vi "FRCts20_WebMethods_Home_Convert.vi"(8 "error in (no error)":errorcluster, 11 "EventRoot Out":T4) -> (0 "error out":errorcluster, 3 "Events":T1)   [LabVIEW 2014, in "FRCts20_WebMethods.lvlib"]
uses:
  FRCts20_WebMethods.lvlib
  Web Method Public Interface/FRCts20_WebMethods_ctl_teamIdentifier.ctl
  Web Method Public Interface/FRCts20_WebMethods_ctl_singleEvent.ctl
  Web Method Public Interface/FRCts20_WebMethods_ctl_events.ctl
  Backend/source/VI Source/FRCts20_Backend_API/FRCts20_Backend_API_EventRoot.ctl
  Backend/source/VI Source/FRCts20_Backend_API/FRCts20_Backend_API.lvlib
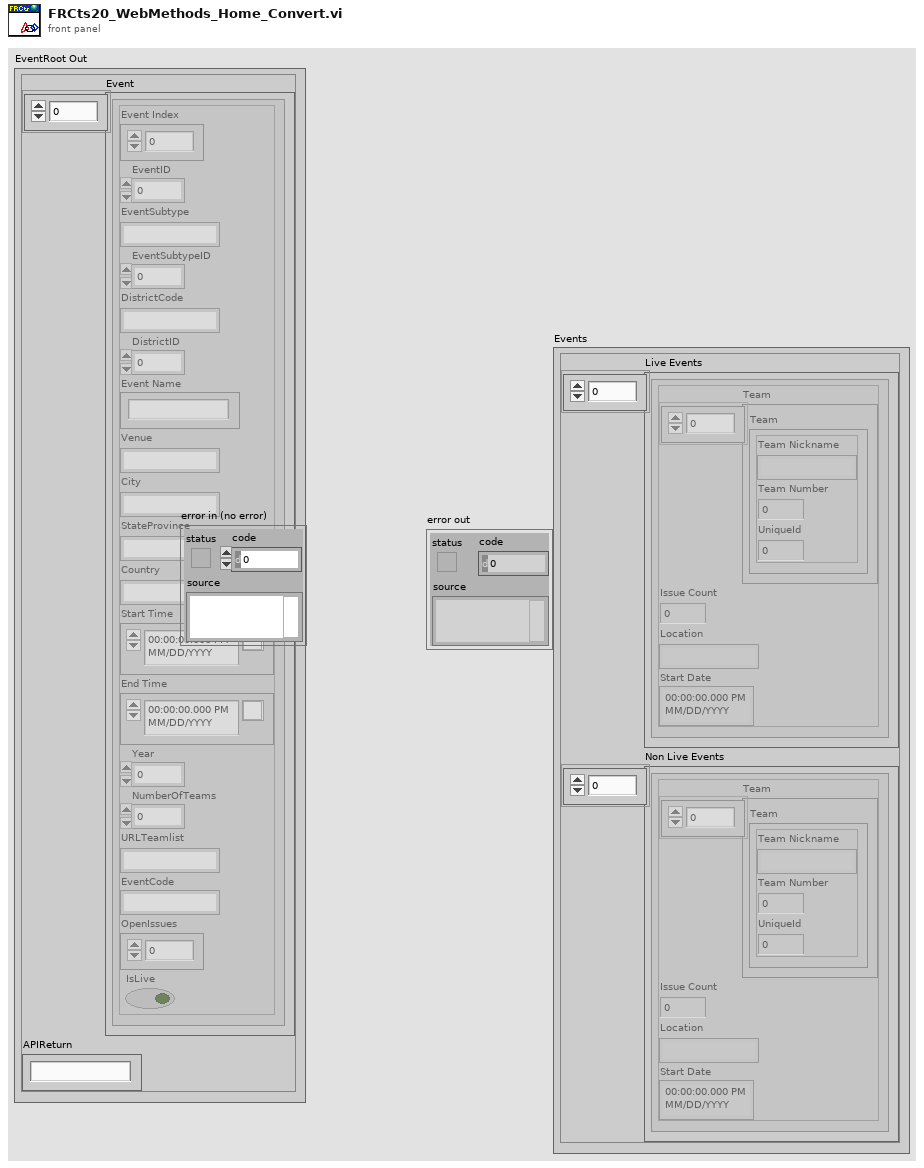
[diagram p1: front panel]
types:
  T1 = typedef "FRCts20_WebMethods.lvlib/FRCts20_WebMethods_ctl_events.ctl" = cluster{"Live Events":cluster{"Team":T2[], "Issue Count":i32, "Location":string, "Start Date ":timestamp}[], "Non Live Events":T3[]}
  T2 = typedef "FRCts20_WebMethods.lvlib/FRCts20_WebMethods_ctl_teamIdentifier.ctl" = cluster{"Team Nickname":string, "Team Number ":u32, "UniqueId":u32}
  T3 = typedef "FRCts20_WebMethods.lvlib/FRCts20_WebMethods_ctl_singleEvent.ctl" = cluster{"Team":T2[], "Issue Count":i32, "Location":string, "Start Date ":timestamp}
  T4 = typedef "FRCts20_Backend_API.lvlib/FRCts20_Backend_API_EventRoot.ctl" = cluster{"Event":cluster{"Event Index":u32, "EventID":u32, "EventSubtype":string, "EventSubtypeID":u32, "DistrictCode":string, "DistrictID":u32, "Event Name":string, "Venue":string, "City":string, "StateProvince":string, "Country":string, "Start Time":timestamp, "End Time":timestamp, "Year":u32, "NumberOfTeams":u32, "URLTeamlist":string, "EventCode":string, "OpenIssues":u8, "IsLive":bool}[], "APIReturn":string}
  T5 = cluster{"Team":T2[], "Issue Count":i32, "Location":string, "Start Date ":timestamp}
  T6 = cluster{"Event Index":u32, "EventID":u32, "EventSubtype":string, "EventSubtypeID":u32, "DistrictCode":string, "DistrictID":u32, "Event Name":string, "Venue":string, "City":string, "StateProvince":string, "Country":string, "Start Time":timestamp, "End Time":timestamp, "Year":u32, "NumberOfTeams":u32, "URLTeamlist":string, "EventCode":string, "OpenIssues":u8, "IsLive":bool}[]
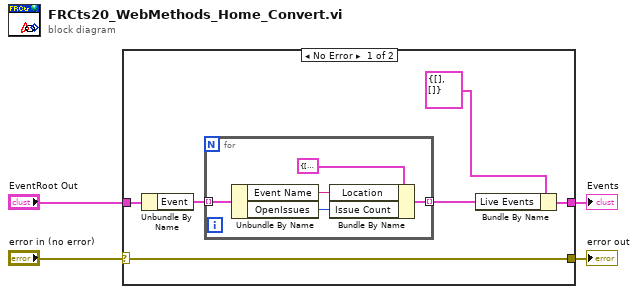
[diagram p0: block diagram]
diagram:
  n1 = case shown="No Error" "error in (no error)" {
    selector: "error in (no error)" -> [w5 w16]
    tunnel: [w5 w16] -> w4
    tunnel: "EventRoot Out" -> [w10 _]
    tunnel: [w6 _] -> w1
    frame No Error {
      n2 = Unbundle By Name(w10) -> ("Event"=w8:T6)
      n3 = for {
        tunnel: w8 -> [w15] mode=indexing
        tunnel: [w11] -> w7 mode=indexing
        n4 = Unbundle By Name(w15) -> ("Event Name"=w13:string, "OpenIssues"=w14:u8)
        n5 = Bundle By Name(cluster=T5 {"Team"=[], "Issue Count"=0, "Location"="", "Start Date "=timestamp(0 s since 1904-01-01)} ("Single Event"), "Location"=w13, "Issue Count"=w14) -> (w11:T5)
      }
      n6 = Bundle By Name(cluster=T1 {"Live Events"=[], "Non Live Events"=[]} ("Events"), "Live Events"=w7) -> (w6:T1)
    }
    frame Error {
    }
  }
  "error out" <- w4
  "Events" <- w1
